vi "TP 2.3.vi"() -> ()   [LabVIEW 2013]
panel:
  in  "Boolean":bool
  in  "stop":bool
  out "Waveform Graph":dbl[](graph)
  in  "Amplitud":dbl
  in  "Frecuencia":dbl
  in  "Cantida de Muestras":dbl
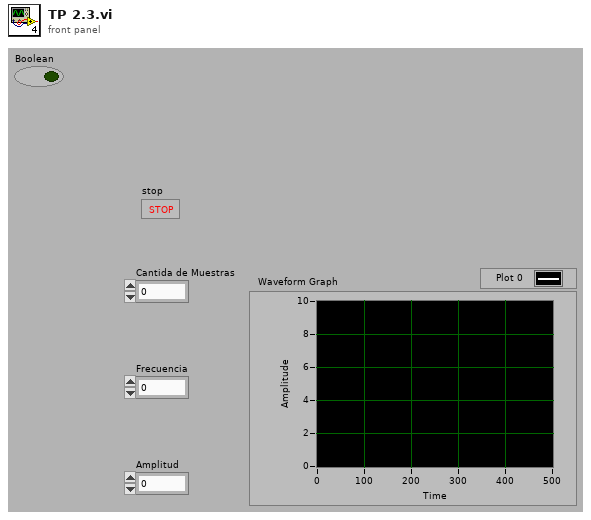
[diagram p1: front panel]
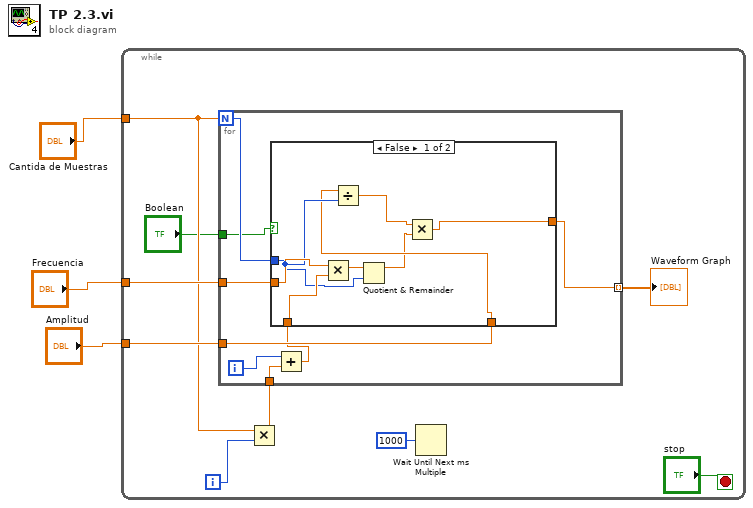
[diagram p0: block diagram]
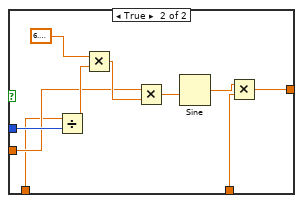
[diagram p2: hidden frame]
diagram:
  n1 = while {
    tunnel: "Cantida de Muestras" -> [w6]
    tunnel: "Frecuencia" -> [w12]
    tunnel: "Amplitud" -> [w11]
    i -> [w7]
    stop <- "stop" stop-if-true
    n2 = Multiply(x=w6, y=w7) -> (x*y=w5:dbl)
    n3 = for {
      N: w6 -> [w20]
      tunnel: w12 -> [w19]
      tunnel: w11 -> [w18]
      tunnel: [w17] -> w10 mode=indexing
      tunnel: w5 -> [w16]
      tunnel: "Boolean" -> [w13]
      i -> [w15]
      n4 = Add(x=w15, y=w16) -> (x+y=w14:dbl)
      n5 = case shown="False" w13 {
        tunnel: w20 -> [w25 w38]
        tunnel: w19 -> [w27 w35]
        tunnel: w18 -> [w24 w31]
        tunnel: [w21 w30] -> w17
        tunnel: w14 -> [w28 w29]
        frame False {
          n6 = Multiply(x=w27, y=w28) -> (x*y=w26:dbl)
          n7 = Divide(x=w24, y=w25) -> (x/y=w23:dbl)
          n8 = Quotient & Remainder(x=w26, y=w25) -> (x-y*floor(x/y)=w22:dbl)  [unwired: 1 out]
          n9 = Multiply(x=w23, y=w22) -> (x*y=w21:dbl)
        }
        frame True {
          n10 = Divide(x=w29, y=w38) -> (x/y=w37:dbl)
          n11 = Multiply(x=6.283185307179586, y=w37) -> (x*y=w36:dbl)
          n12 = Multiply(x=w35, y=w36) -> (x*y=w33:dbl)
          n13 = Sine(x=w33) -> (sin(x)=w32:dbl)
          n14 = Multiply(x=w32, y=w31) -> (x*y=w30:dbl)
        }
      }
    }
    "Waveform Graph" <- w10
    n15 = Wait Until Next ms Multiple(millisecond multiple=u32 1000) -> ()  [unwired: 1 out]
  }
